vi "Enqueue Message (several exceptions same to all queues).vi"(6 "Priority":bool, 7 "Exclude":string[](array[string]), 8 "error in (no error)":errorcluster, 9 "Message Data Array":variant[](array[variant]), 10 "Message":string, 11 "Message Queues in":T1) -> (0 "error out":errorcluster, 3 "Message Queues out":T1)   [LabVIEW 2017, in "Message Queue.lvlib"]
uses:
  Message Queue.lvlib
  All Message Queues.ctl
  Message Cluster.ctl
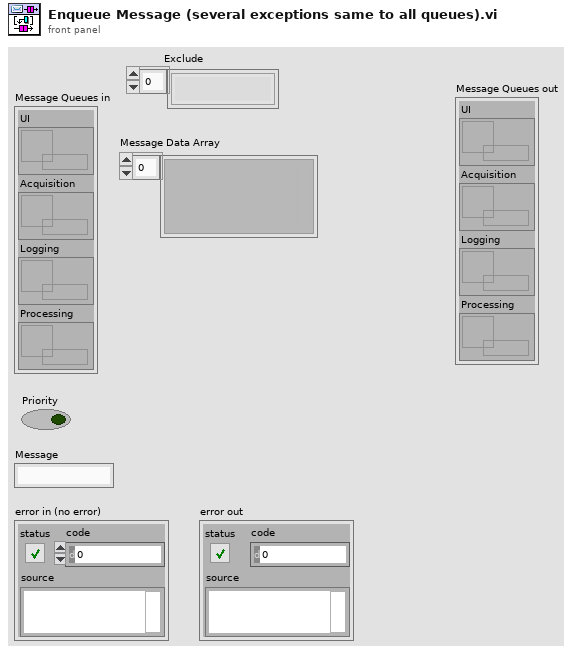
[diagram p1: front panel]
types:
  T1 = typedef "Message Queue.lvlib/All Message Queues.ctl" = cluster{"UI":refnum<queue>, "Acquisition":refnum<queue>, "Logging":refnum<queue>, "Processing":refnum<queue>}
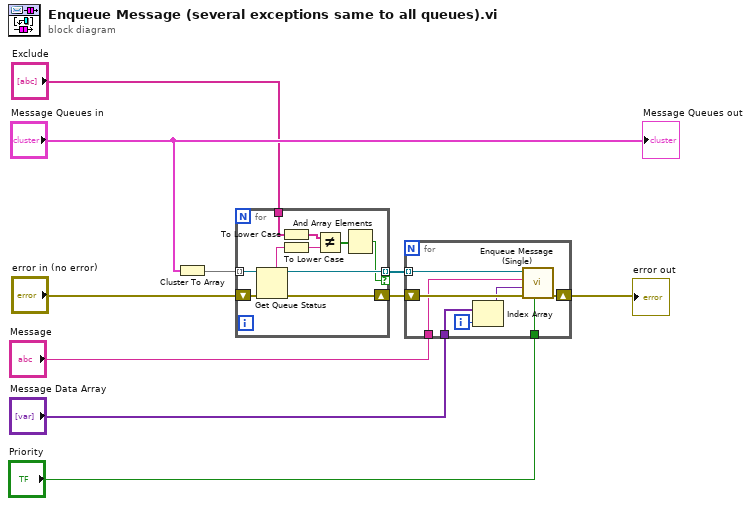
[diagram p0: block diagram]
diagram:
  n1 = Cluster To Array(cluster="Message Queues in") -> (array=w7:refnum<queue>[])
  n2 = for {
    tunnel: w7 -> [w20] mode=indexing
    tunnel: [w19] -> w8 mode=indexing if=w11
    shift-right: [w18] -> w9
    shift-left: "error in (no error)" -> [w17]
    tunnel: "Exclude" -> [w13]
    n3 = Get Queue Status(queue=w20, error in (no error)=w17) -> (queue out=w19:refnum<queue>, queue name=w16:string, error out=w18:errorcluster)  [unwired: 1 in, 5 out]
    n4 = To Lower Case(string=w13) -> (all lower case string=w14:string[])
    n5 = To Lower Case(string=w16) -> (all lower case string=w15:string)
    n6 = Not Equal?(x=w14, y=w15) -> (x != y?=w12:bool[])
    n7 = And Array Elements(Boolean array=w12) -> (logical AND=w11:bool)
  }
  n8 = for {
    shift-right: [w27] -> w5
    shift-left: w9 -> [w28]
    tunnel: w8 -> [w26] mode=indexing
    tunnel: "Message" -> [w25]
    tunnel: "Priority" -> [w24]
    tunnel: "Message Data Array" -> [w21]
    i -> [w22]
    n9 = Index Array(array=w21, index=w22) -> (element=w23:variant)
    n10 = call "Enqueue Message (Single).vi"("Priority Message? (F)"=w24, "error in (no error)"=w28, "Message Data"=w23, "Message"=w25, "Message Queue"=w26) -> ("error out"=w27:errorcluster)  [unwired: 5 in, 1 out]
  }
  "error out" <- w5
  "Message Queues out" <- "Message Queues in"
